vi "CPP_Aeroprobe_dT-Unified.vi"() -> (5 "Plug in titles":string[](array[string]), 7 "Plug in values":string[](array[string]))   [LabVIEW 2013]
uses:
  Globals/Meas_global.vi
panel:
  in  "Graphs":bool=TRUE
  in  "Downsampler":i32=10
  in  "Calibration Folder Path":path=path "G:/5HoleProbe"
  in  "Correction File Path":path=path "M:/Preferences/Rig_Setups/All_Rigs/TubingCompensation/5HPTubingCorrection12066.xls"
  in  "Apply Phase Correction?":bool=TRUE
  out "Zeroes":dbl[](array[numeric])
  # "!! 5-hole 1-5 must be connected to Channels 1-5 !!"
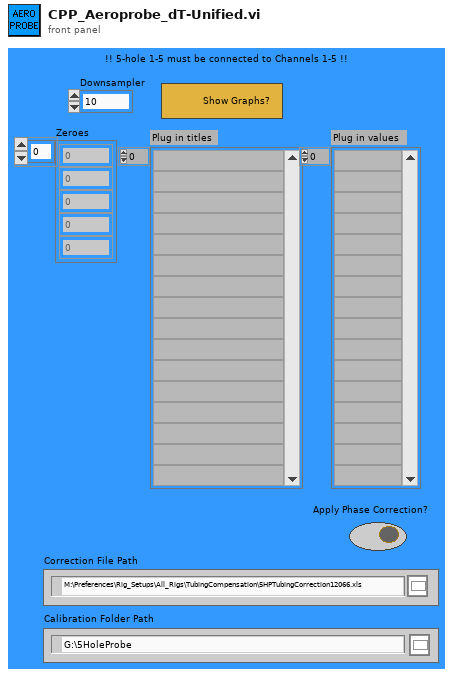
[diagram p1: front panel]
types:
  T1 = typedef "Analysis_info_cluster.ctl" = cluster{"Colour":u32, "Inst type":T2, "Inst name":string, "Symbol":string, "Code name":string, "Extra Info":string, "Inst Array":T3, "Extra Titles":string[], "Extra Values":string[], "U":dbl, "u^2":dbl, "u^3":dbl, "u^4":dbl, "Skew_u":dbl, "Kurt_u":dbl, "Sd Error in Mean":dbl, "% u'/U":dbl, "X":dbl, "Y":dbl, "Z":dbl, "Timescale integral to 25%":dbl, "Sd Error in Variance":dbl, "Calib File":path, "Calib Constants":dbl[], "Output Position":bool, "Full Stats":bool, "Av Sampling Rate":dbl, "Av No of Samples":dbl, "Total Meas Time (s)":dbl, "ADAM Ch Name":string}
  T2 = typedef "Inst_type.ctl" = enum16{"Propeller anemometer", "Raw voltage", "Pressure Transducer", "Pitot-static tube", "Preston tube", "Hot wire", "Cross wire 1", "Cross wire 2", "Generic Linear", "Generic Polynomial", "Generic BackPoly", "Fast FID", "Thermocouple", "Cold wire", "Pulsed Wire", "LDA Vel", "LDA Tran time", "LDA Arr time"}
  T3 = typedef "Instrument_Array.ctl" = enum16{"PWA", "LDA", "Analogue"}
  T4 = cluster{"Analysis Info cluster[0]":T1, "Analysis Info cluster[1]":T1, "Analysis Info cluster[2]":T1, "Analysis Info cluster[3]":T1, "Analysis Info cluster[4]":T1, "Analysis Info cluster[5]":T1, "Analysis Info cluster[6]":T1}
  T5 = typedef "Time_Trace_Cluster.ctl" = cluster{"Weighting":dbl[], "Time (s)":dbl[], "Voltage":dbl[], "Eng Values":dbl[]}
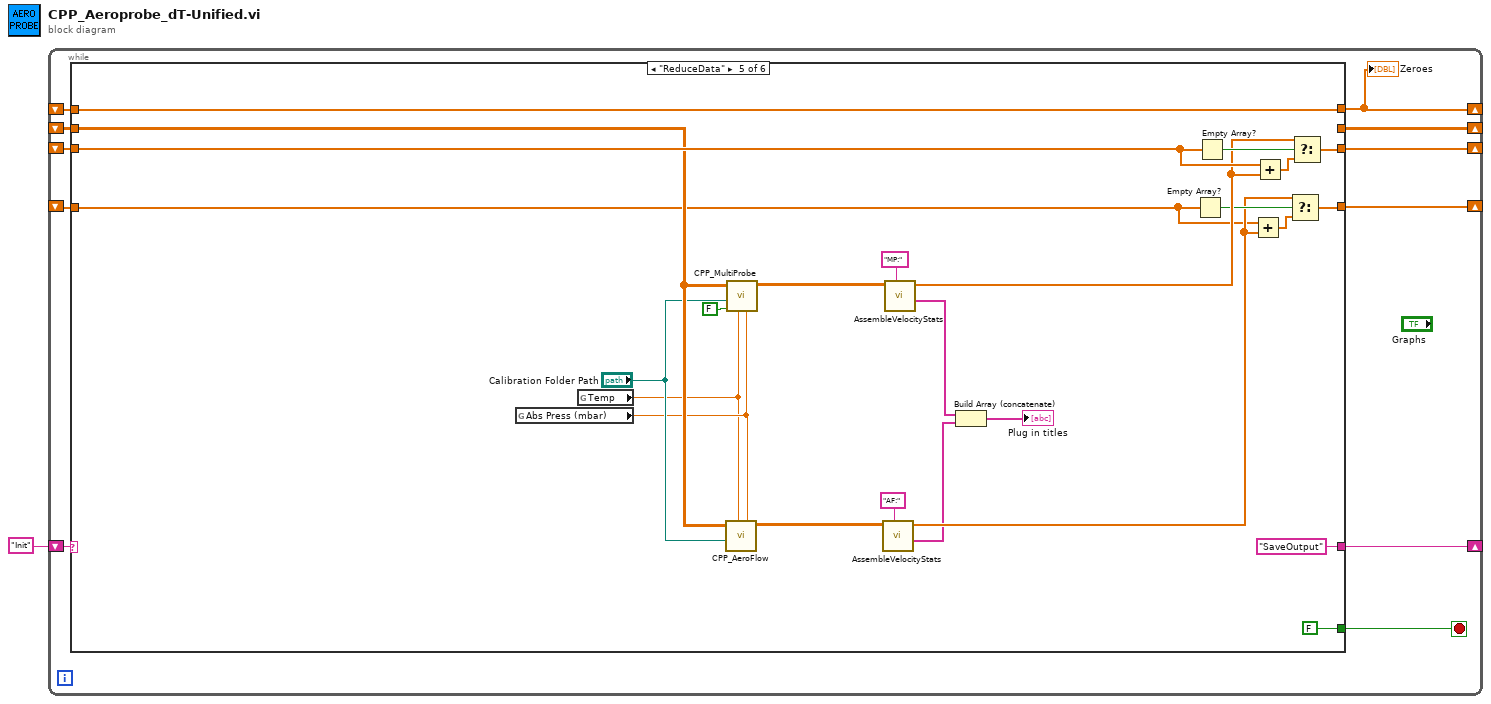
[diagram p0: block diagram]
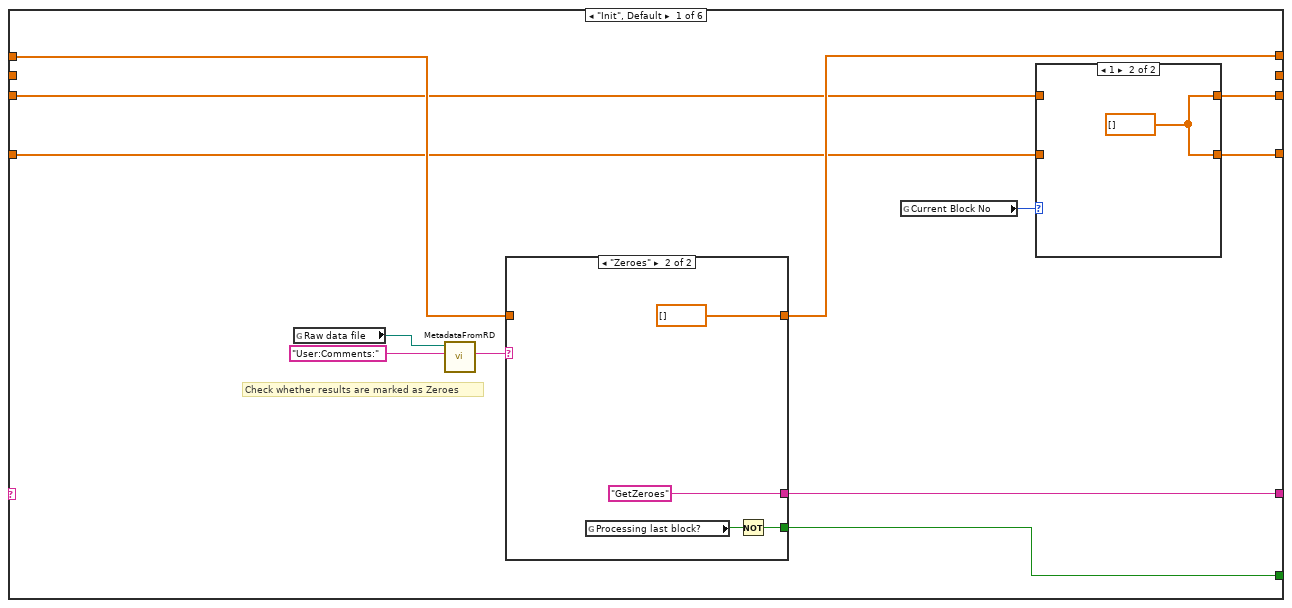
[diagram p2: hidden frame]
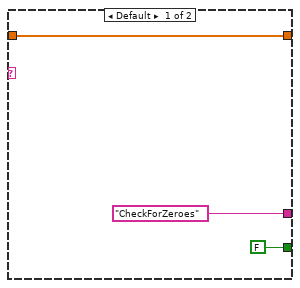
[diagram p4: hidden frame]
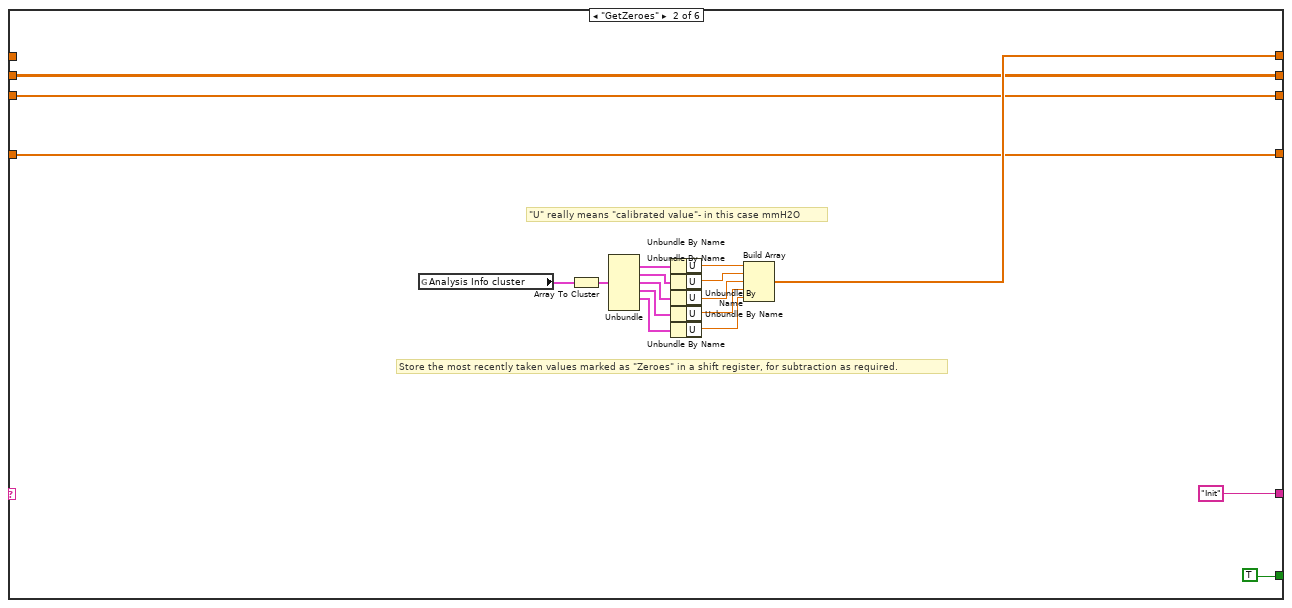
[diagram p5: hidden frame]
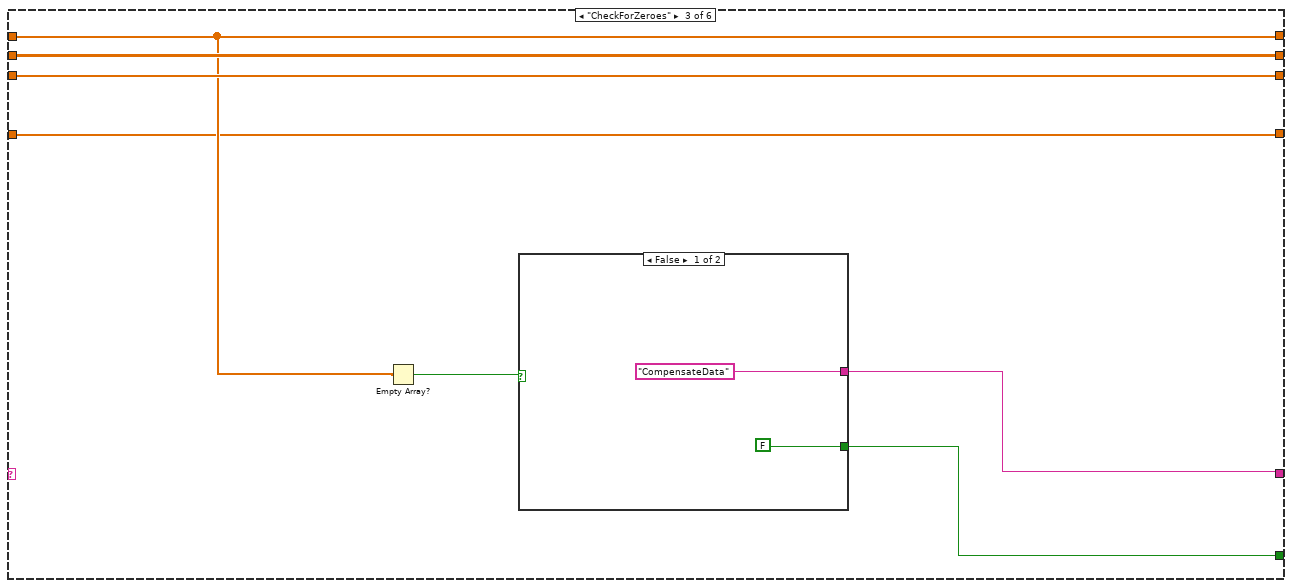
[diagram p6: hidden frame]
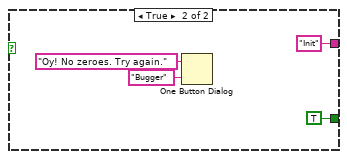
[diagram p7: hidden frame]
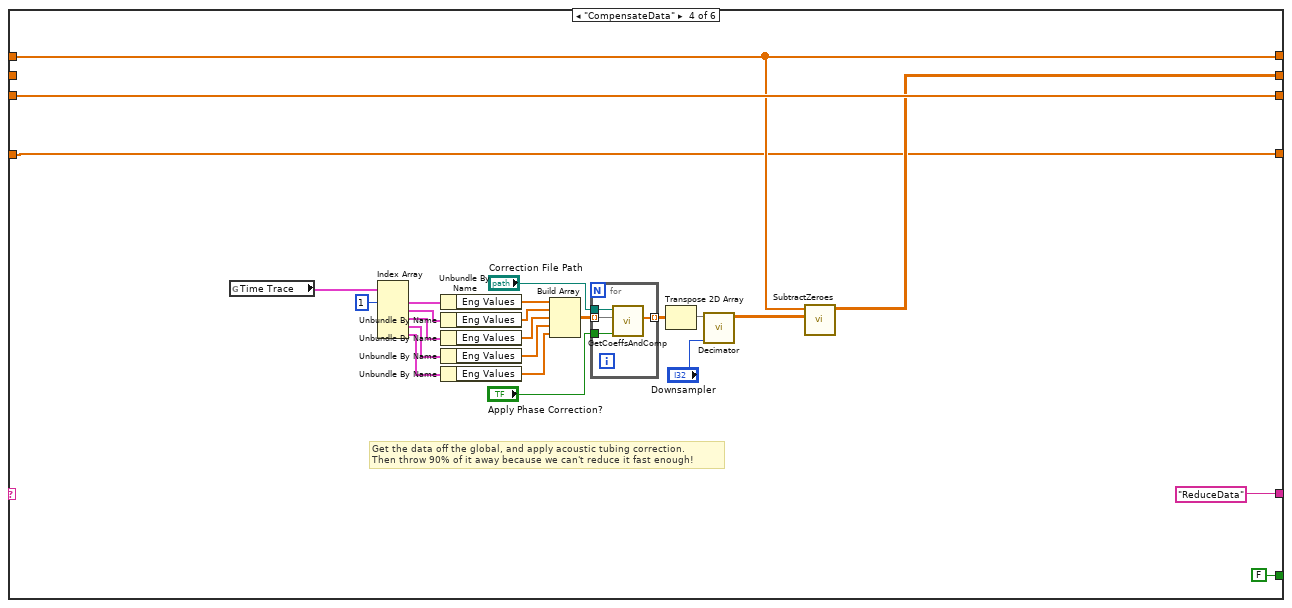
[diagram p8: hidden frame]
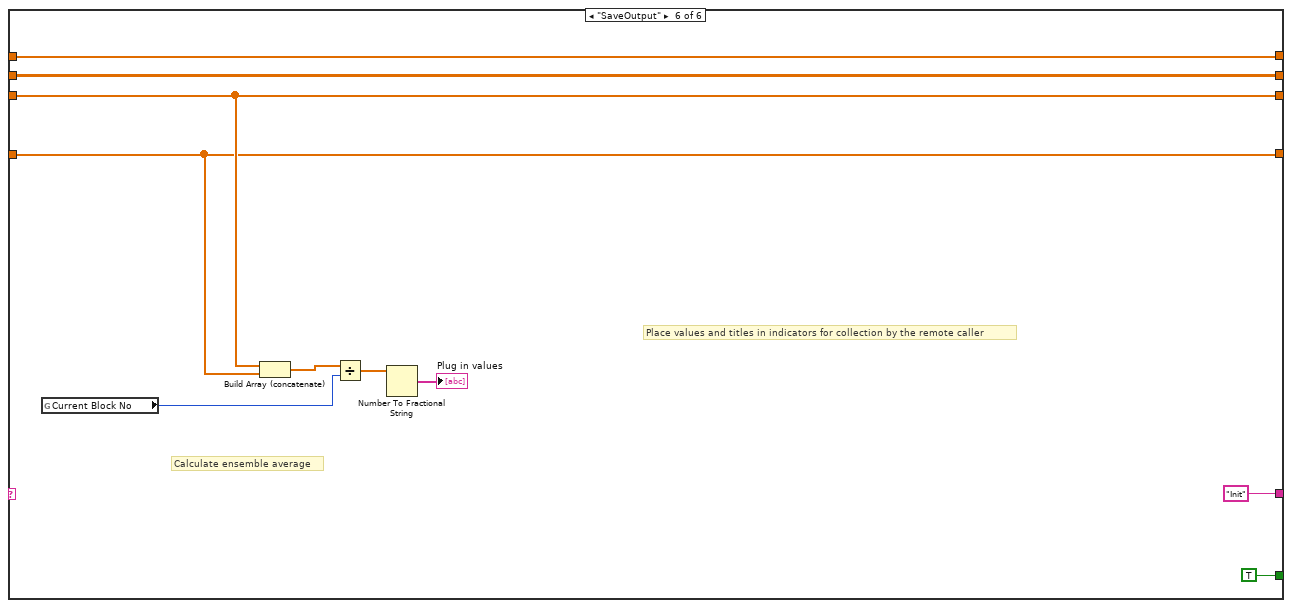
[diagram p9: hidden frame]
diagram:
  n1 = while {
    shift-right: [w11] -> _
    shift-left: "Init" -> [w12]
    shift-right: [w10] -> _
    shift-left: _ -> [w9]
    shift-right: [w8] -> _
    shift-left: _ -> [w7]
    shift-right: [w5] -> _
    shift-left: _ -> [w4]
    shift-right: [w3] -> _
    shift-left: _ -> [w2]
    stop <- w6 stop-if-true
    n2 = case shown="\"ReduceData\"" w12 {
      tunnel: [w24 "Init" w58 "ReduceData" "SaveOutput" "Init"] -> w11
      tunnel: [w18 w39 w55 w70 w118 w129] -> w10
      tunnel: w9 -> [w19 _ w55 w70 w118 w129]
      tunnel: [w17 w37 w59 w90 w113 w124] -> w8
      tunnel: w7 -> [w16 w37 w59 w90 w116 w124]
      tunnel: [w20 TRUE w57 FALSE FALSE TRUE] -> w6
      tunnel: [_ w36 w56 w69 _ w123] -> w5
      tunnel: w4 -> [_ w36 w56 _ w109 w123]
      tunnel: [w14 w35 w53 w67 w103 w120] -> w3
      tunnel: w2 -> [w13 w35 w53 w67 w101 w120]
      frame "Init", Default {
        # "Check whether results are marked as Zeroes"
        n3 = global read "Meas_global.vi" "Raw data file"() -> (w23:path)
        n4 = call "MetadataFromRD.vi"("ChannelName"="User:Comments:", "Raw data file"=w23) -> ("ValueString"=w21:string)  [unwired: 8 in, 1 out]
        n5 = case shown="\"Zeroes\"" w21 {
          tunnel: ["CheckForZeroes" "GetZeroes"] -> w24
          tunnel: [FALSE w33] -> w20
          tunnel: w19 -> [w28 _]
          tunnel: [w28 dbl[] [] ("t")] -> w18
          frame Default {
          }
          frame "Zeroes" {
            n6 = global read "Meas_global.vi" "Processing last block?"() -> (w32:bool)
            n7 = Not(x=w32) -> (.not. x?=w33:bool)
          }
        }
        n8 = global read "Meas_global.vi" "Current Block No"() -> (w15:i32)
        n9 = case shown="1" w15 {
          tunnel: [w26 w27] -> w17
          tunnel: w16 -> [w26 _]
          tunnel: [w25 w27] -> w14
          tunnel: w13 -> [w25 _]
          frame 0, Default {
          }
          frame 1 {
            w27 = dbl[] [] ("t")
          }
        }
      }
      frame "GetZeroes" {
        # "Store the most recently taken values marked as \"Zeroes\" in a shift register, for subtraction as required."
        # "\"U\" really means \"calibrated value\"- in this case mmH2O"
        n10 = global read "Meas_global.vi" "Analysis Info cluster"() -> (w41:T1[])
        n11 = Array To Cluster(array=w41) -> (cluster=w47:T4)
        n12 = Unbundle(w47) -> ("Analysis Info cluster[1]"=w48:T1, "Analysis Info cluster[2]"=w49:T1, "Analysis Info cluster[3]"=w50:T1, "Analysis Info cluster[4]"=w51:T1, "Analysis Info cluster[5]"=w52:T1)  [unwired: 2 out]
        n13 = Unbundle By Name(w48) -> ("U"=w46:dbl)
        n14 = Unbundle By Name(w49) -> ("U"=w45:dbl)
        n15 = Unbundle By Name(w50) -> ("U"=w44:dbl)
        n16 = Unbundle By Name(w51) -> ("U"=w43:dbl)
        n17 = Unbundle By Name(w52) -> ("U"=w42:dbl)
        n18 = Build Array(w46, w45, w44, w43, w42) -> (w39:dbl[])
      }
      frame "CheckForZeroes" {
        n19 = Empty Array?(array=w55) -> (empty?=w54:bool)
        n20 = case shown="False" w54 {
          tunnel: ["CompensateData" "Init"] -> w58
          tunnel: [FALSE TRUE] -> w57
          frame False {
          }
          frame True {
            n21 = One Button Dialog(message="Oy! No zeroes. Try again.", button name ("OK")="Bugger") -> ()  [unwired: 1 out]
          }
        }
      }
      frame "CompensateData" {
        # "Get the data off the global, and apply acoustic tubing correction. \nThen throw 90% of it away because we can't reduce it fast enough!"
        n22 = global read "Meas_global.vi" "Time Trace"() -> (w80:T5[])
        n23 = Index Array(array=w80, index #1=1 ("index")) -> (element #1=w79:T5, element #2=w88:T5, element #3=w87:T5, element #4=w86:T5, element #5=w85:T5)  [unwired: 4 in]
        n24 = Unbundle By Name(w79) -> ("Eng Values"=w78:dbl[])
        n25 = Unbundle By Name(w88) -> ("Eng Values"=w84:dbl[])
        n26 = Unbundle By Name(w87) -> ("Eng Values"=w83:dbl[])
        n27 = Unbundle By Name(w86) -> ("Eng Values"=w82:dbl[])
        n28 = Unbundle By Name(w85) -> ("Eng Values"=w81:dbl[])
        n29 = Build Array(w78, w84, w83, w82, w81) -> (w77:dbl[][])
        n30 = for {
          tunnel: w77 -> [w94] mode=indexing
          tunnel: [w93] -> w74 mode=indexing
          tunnel: "Apply Phase Correction?" -> [w92]
          tunnel: "Correction File Path" -> [w91]
          n31 = call "GetCoeffsAndComp.vi"("Apply Phase Correction?"=w92, "mutedData"=w94, "TubingCorrectionFile"=w91) -> ("boostedData"=w93:dbl[])  [unwired: 8 in]
        }
        n32 = Transpose 2D Array(2D array=w74) -> (transposed array=w73:dbl[][])
        n33 = call "Decimator.vi"("Decimator"="Downsampler", "Array In"=w73) -> ("DecimatedArrayOut"=w71:dbl[][])  [unwired: 9 in]
        n34 = call "SubtractZeroes.vi"("RawPressure"=w71, "Zeroes"=w70) -> ("ZeroedPressure"=w69:dbl[][])  [unwired: 9 in]
      }
      frame "ReduceData" {
        n35 = global read "Meas_global.vi" "Abs Press (mbar)"() -> (w107:dbl)
        n36 = global read "Meas_global.vi" "Temp"() -> (w106:dbl)
        n37 = call "CPP_AeroFlow.vi"("Pressure (mBar)"=w107, "Temperature (C)"=w106, "Calibration Folder Path"="Calibration Folder Path", "ZeroedPressures (mmH2O)"=w109) -> ("RawVmagUVWCone"=w110:dbl[][])  [unwired: 2 in, 3 out]
        n38 = call "CPP_MultiProbe.vi"("Pressure (mBar)"=w107, "Temperature (C)"=w106, "Old5HoleProbe?"=FALSE, "Calibration Folder Path"="Calibration Folder Path", "ZeroedPressures (mmH2O)"=w109) -> ("RawVmagUVWCone"=w111:dbl[][])  [unwired: 1 in, 3 out]
        n39 = call "AssembleVelocityStats.vi"("TitlePrefix"="AF:", "VmagUVWCone"=w110) -> ("Plug in titles"=w97:string[], "StatsArray"=w102:dbl[])  [unwired: 8 in]
        n40 = call "AssembleVelocityStats.vi"("TitlePrefix"="MP:", "VmagUVWCone"=w111) -> ("Plug in titles"=w96:string[], "StatsArray"=w112:dbl[])  [unwired: 8 in]
        n41 = Build Array (concatenate)(w96, w97) -> (→"Plug in titles":string[])
        n42 = Empty Array?(array=w101) -> (empty?=w104:bool)
        n43 = Empty Array?(array=w116) -> (empty?=w115:bool)
        n44 = Add(x=w101, y=w102) -> (x+y=w105:dbl[])
        n45 = Add(x=w116, y=w112) -> (x+y=w114:dbl[])
        n46 = Select(t=w102, s=w104, f=w105) -> (s? t:f=w103:dbl[])
        n47 = Select(t=w112, s=w115, f=w114) -> (s? t:f=w113:dbl[])
      }
      frame "SaveOutput" {
        # "Place values and titles in indicators for collection by the remote caller"
        # "Calculate ensemble average"
        n48 = global read "Meas_global.vi" "Current Block No"() -> (w125:i32)
        n49 = Build Array (concatenate)(w124, w120) -> (w121:dbl[])
        n50 = Divide(x=w121, y=w125) -> (x/y=w122:dbl[])
        n51 = Number To Fractional String(number=w122) -> (F-format string=→"Plug in values":string[])  [unwired: 3 in]
      }
    }
    "Zeroes" <- w10
  }
